vi "Set Target Temp.vi"(5 "Temp Chan":string, 7 "T Set":dbl, 8 "error in (no error)":errorcluster, 11 "IP Address in":string) -> (0 "error out":errorcluster)   [LabVIEW 2018]
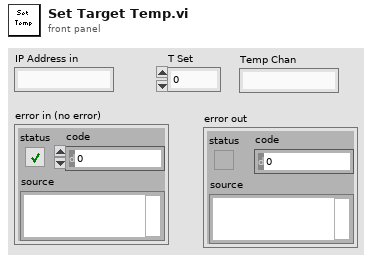
[diagram p1: front panel]
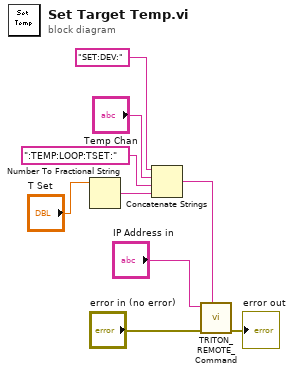
[diagram p0: block diagram]
diagram:
  n1 = Number To Fractional String(number="T Set") -> (F-format string=w4:string)  [unwired: 3 in]
  n2 = Concatenate Strings("SET:DEV:" ("string"), "Temp Chan", ":TEMP:LOOP:TSET:" ("Command to send"), w4) -> (w3:string)
  n3 = call "TRITON_REMOTE_Command.vi"("Command to send"=w3, "error in (no error)"="error in (no error)", "IP Address"="IP Address in") -> ("error out"=→"error out":errorcluster)  [unwired: 6 in, 2 out]
